vi "find first peak - amplitude (SubVI).vi"(6 "Noise duration (units)":i32=5, 8 "Noise min (amplitude)":dbl format="%0.2f", 9 "threshold ratio":dbl=3.0, 10 "peak width (units)":i32=3, 11 "Array":dbl[](array[numeric])) -> (0 "Peak threshold":dbl, 1 "noise index":dbl[](array[numeric]), 2 "peak amplitude":dbl, 3 "Index":dbl, 4 "#peaks":i32)   [LabVIEW 2018]
uses:
  <vilib>/Analysis/NI_AAL_SigProc.lvlib
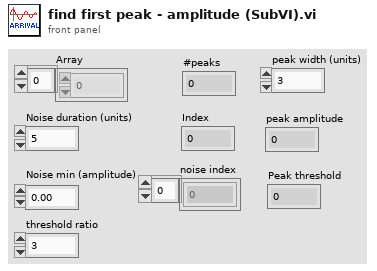
[diagram p1: front panel]
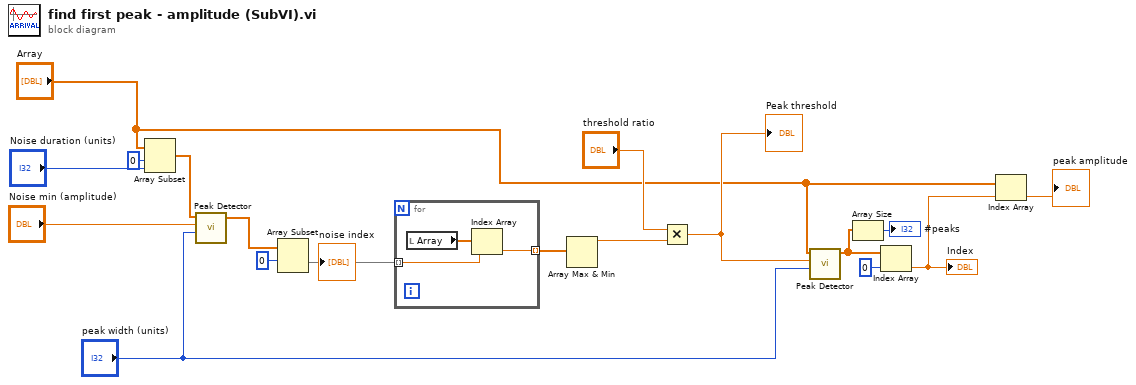
[diagram p0: block diagram]
diagram:
  n1 = Array Subset(array="Array", index=0, length="Noise duration (units)") -> (w3:dbl[])
  n2 = call <vilib>:"Peak Detector.vi"("width"="peak width (units)", "threshold"="Noise min (amplitude)", "X"=w3) -> ("Locations"=w11:dbl[])  [unwired: 4 in, 4 out]
  n3 = Array Subset(array=w11, index=0) -> (w9:dbl[])  [unwired: 1 in]
  "noise index" <- w9
  n4 = for {
    tunnel: w9 -> [w21] mode=indexing
    tunnel: [w19] -> w8 mode=indexing
    n5 = local read "Array"() -> (w20:dbl[])
    n6 = Index Array(array=w20, index=w21) -> (element=w19:dbl)
  }
  n7 = Array Max & Min(array=w8) -> (max value=w7:dbl)  [unwired: 3 out]
  n8 = Multiply(x="threshold ratio", y=w7) -> (x*y=w6:dbl)
  "Peak threshold" <- w6
  n9 = call <vilib>:"Peak Detector.vi"("width"="peak width (units)", "threshold"=w6, "X"="Array") -> ("Locations"=w16:dbl[])  [unwired: 4 in, 4 out]
  n10 = Array Size(array=w16) -> (size(s)=→"#peaks":i32)
  n11 = Index Array(array=w16, index=0) -> (element=w15:dbl)
  "Index" <- w15
  n12 = Index Array(array="Array", index=w15) -> (element=→"peak amplitude":dbl)
